vi "InitAction.vi"(6 "InstrumentName":string, 7 "VisaRessIn":refnum<visa-resource-name>, 8 "error in (no error)":errorcluster caption="entrée d'erreur (pas d'erreur)", 9 "FirstClassInst":bool, 10 "Function":string, 11 "GenData In":refnum<class "SR830.lvclass"> caption="DNL_LabVIEW Object in") -> (0 "error out":errorcluster caption="sortie d'erreur", 3 "GenData Out":refnum<class "SR830.lvclass"> caption="DNL_LabVIEW Object out")   [LabVIEW 2012, in "SR830.lvclass"]
uses:
  SR830.lvclass
  SR830_Func.ctl
  SR830.lvclass/SR830.ctl
panel:
  in  "DefaultDev_Func":T1
  out "VisaRessOut":refnum<visa-resource-name>
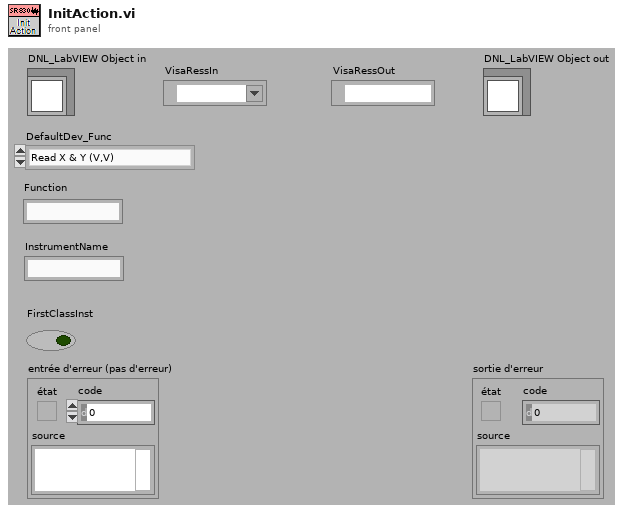
[diagram p1: front panel]
types:
  T1 = typedef "SR830.lvclass/SR830_Func.ctl" = enum16{"Read X & Y (V,V)", "Read Mag & Phase (V,°)", "Read X,Y,Mag & Phase (V,V,V,°)", "Read THz Pump Off/On (V,V,V,°,V,V,V,°,V)"}
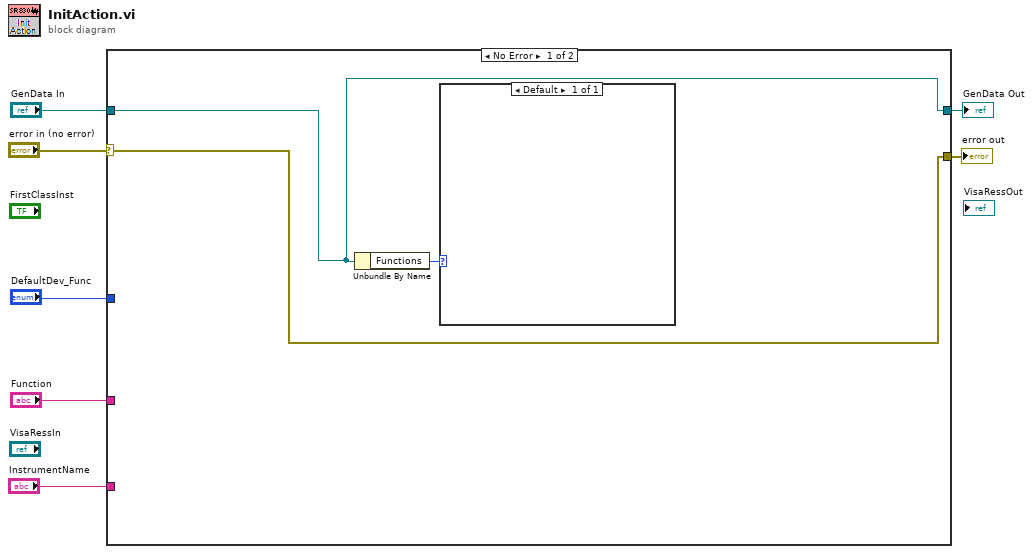
[diagram p0: block diagram]
diagram:
  n1 = case shown="No Error" "error in (no error)" {
    selector: "error in (no error)" -> [w8 w12]
    tunnel: [w8 w12] -> w6
    tunnel: "GenData In" -> [w9 w11]
    tunnel: [w9 w11] -> w4
    tunnel: "DefaultDev_Func" -> [_ _]
    tunnel: "Function" -> [_ _]
    tunnel: "InstrumentName" -> [_ _]
    frame No Error {
      n2 = Unbundle By Name(w9) -> ("Functions"=w10:T1)
      n3 = case shown="Default" w10 {
        frame Default {
        }
      }
    }
    frame Error {
    }
  }
  "error out" <- w6
  "GenData Out" <- w4
